vi "resize.navigation.pane.vi"(8 "error in (no error)":errorcluster, 11 "vi ref":refnum<vi>) -> (0 "error out":errorcluster)   [LabVIEW 2024]
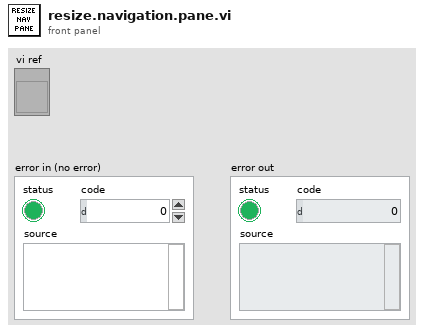
[diagram p1: front panel]
types:
  T1 = map{string, cluster{"offset":i32, "position":enum16{"left", "center", "right"}}}
  T2 = cluster{"offset":i32, "position":enum16{"left", "center", "right"}}
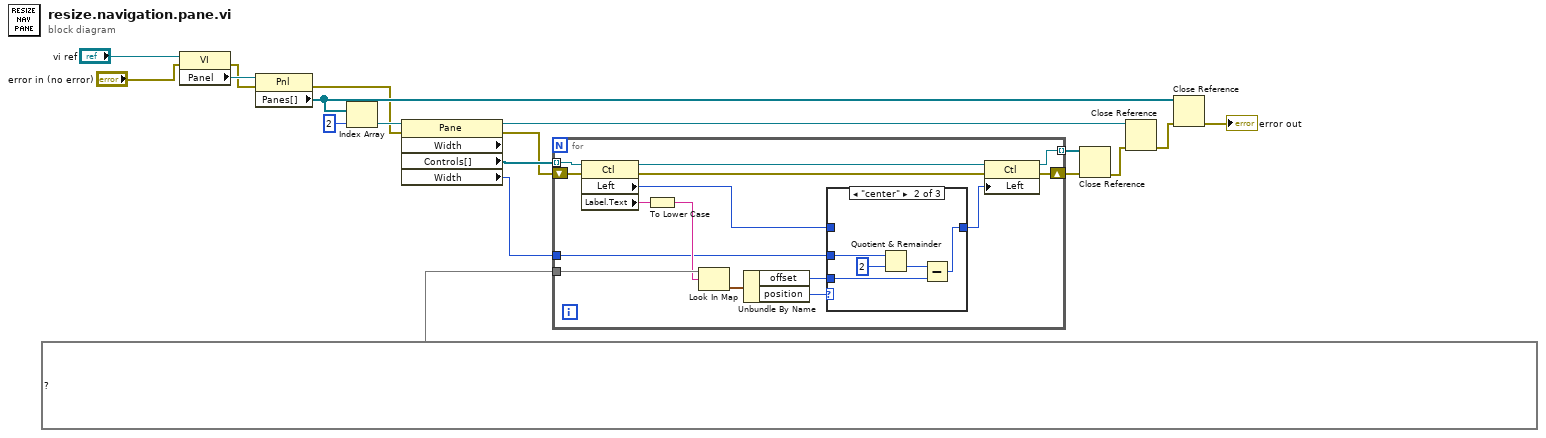
[diagram p0: block diagram]
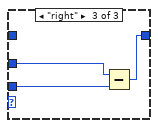
[diagram p3: hidden frame]
diagram:
  n1 = property class="VI"(reference="vi ref", error in="error in (no error)") -> (error out=w17:errorcluster, "Panel"=w18:refnum<vi>)  [unwired: 1 out]
  n2 = property class="Pnl"(reference=w18, error in=w17) -> (error out=w1:errorcluster, "Panes[]"=w6:refnum<vi>[])  [unwired: 1 out]
  n3 = Index Array(array=w6, index=2) -> (element=w13:refnum<vi>)
  n4 = property class="Pane" props=["Width", "Controls[]", "Width"](reference=w13, error in=w1) -> (reference out=w7:refnum<vi>, error out=w11:errorcluster, "Controls[]"=w12:refnum<vi>[], "Width"=w2:u32)  [unwired: 1 out]
  n5 = for {
    tunnel: w12 -> [w33] mode=indexing
    shift-right: [w20] -> w9
    shift-left: w11 -> [w32]
    tunnel: [w19] -> w10 mode=indexing
    tunnel: T1 {"dec end"={"offset"=119, "position"=enum."right"}, "dec start"={"offset"=7, "position"=enum."left"}, "dec time"={"offset"=44, "position"=enum."center"}, "inc end"={"offset"=63, "position"=enum."right"}, "inc start"={"offset"=67, "position"=enum."left"}, "inc time"={"offset"=-4, "position"=enum."center"}, "plot end"={"offset"=135, "position"=enum."right"}, "plot start"={"offset"=8, "position"=enum."left"}, "show legend"={"offset"=120, "position"=enum."left"}, "step size"={"offset"=-68, "position"=enum."center"}, "volume"={"offset"=294, "position"=enum."center"}} ("map") -> [w31]
    tunnel: w2 -> [w26]
    n6 = property class="Ctl"(reference=w33, error in=w32) -> (reference out=w21:refnum<vi>, error out=w22:errorcluster, "Left"=w25:i32, "Label.Text"=w30:string)
    n7 = To Lower Case(string=w30) -> (all lower case string=w29:string)
    n8 = Look In Map(map=w31, key=w29) -> (value=w28:T2)  [unwired: 1 in, 1 out]
    n9 = Unbundle By Name(w28) -> ("offset"=w24:i32, "position"=w27:enum16{"left", "center", "right"})
    n10 = case shown="\"center\"" w27 {
      tunnel: w26 -> [_ w39 w40]
      tunnel: w25 -> [w34 _ _]
      tunnel: [w34 w35 w41] -> w23
      tunnel: w24 -> [_ w36 w42]
      frame "left", Default {
      }
      frame "center" {
        n11 = Quotient & Remainder(x=w39, y=u32 2) -> (floor(x/y)=w37:u32)  [unwired: 1 out]
        n12 = Subtract(x=w37, y=w36) -> (x-y=w35:u32)
      }
      frame "right" {
        n13 = Subtract(x=w40, y=w42) -> (x-y=w41:u32)
      }
    }
    n14 = property class="Ctl"(reference=w21, error in=w22, "Left"=w23) -> (reference out=w19:refnum<vi>, error out=w20:errorcluster)
  }
  n15 = Close Reference(reference=w10, error in (no error)=w9) -> (error out=w8:errorcluster)
  n16 = Close Reference(reference=w7, error in (no error)=w8) -> (error out=w5:errorcluster)
  n17 = Close Reference(reference=w6, error in (no error)=w5) -> (error out=→"error out":errorcluster)
